vi "itc 503 box controller.vi"(6 "Log File Path":path, 7 "itc box action":T3=enum."read sweep table", 8 "error in":errorcluster, 9 "Sweep Table In":dbl[][](array[numeric])=[[650.0, 1334.0, 30.0], [300.0, 1334.0, 0.0], [0.0, 0.0, 0.0], [0.0, 0.0, 0.0], [0.0, 0.0, 0.0], [0.0, 0.0, 0.0], [0.0, 0.0, 0.0], [0.0, 0.0, 0.0], [0.0, 0.0, 0.0], [0.0, 0.0, 0.0], [0.0, 0.0, 0.0], [300.0, 0.0, 0.0], [0.0, 0.0, 0.0], [0.0, 0.0, 0.0], [0.0, 0.0, 0.0], [300.0, 0.0, 0.0]], 10 "input":dbl=300.0, 11 "VISA resource name":refnum<visa-resource-name>="GPIB0::23::INSTR") -> (0 "error out":errorcluster, 1 "Sweep Table":dbl[][](array[numeric])=[[650.0, 1334.0, 30.0], [300.0, 1334.0, 0.0], [0.0, 0.0, 0.0], [0.0, 0.0, 0.0], [0.0, 0.0, 0.0], [0.0, 0.0, 0.0], [0.0, 0.0, 0.0], [0.0, 0.0, 0.0], [0.0, 0.0, 0.0], [0.0, 0.0, 0.0], [0.0, 0.0, 0.0], [300.0, 0.0, 0.0], [0.0, 0.0, 0.0], [0.0, 0.0, 0.0], [0.0, 0.0, 0.0], [300.0, 0.0, 0.0]], 2 "itc box state OUT":T2={"ITC503 Address"="GPIB0::15::INSTR", "ITC temperature"=0.0, "ITC set temperature"=300.0, "heater"=300.0, "gas flow"=1.6, "P"=0.0, "D"=10.0, "I"=0.1, "ITC state"="X0A1C2S01H1L0\r", "nonzero temperature"=0.0, "Magn Field (T)"=0.0})   [LabVIEW 2014]
uses:
  itc 503 box - control.ctl
  itc 503 box state.ctl
  ITC Panel.ctl
  Q - not nan -- real.vi
panel:
  out "F-format string":string
  in  "ITC 503 front panel":T1={"Locked"=FALSE, "Unlocked"=FALSE, "Remote"=FALSE, "Local"=FALSE, "in sweep"=FALSE, "start/stop sweep"=FALSE, "Sweep indicator"="X0A1C2S01H1L0\r", "heater MANUAL"=FALSE, "heater AUTO"=FALSE, "ITC state"="X0A1C2S01H1L0\r", "gas MANUAL"=FALSE, "gas AUTO"=FALSE, "heater"=13.5, "gas flow %"=0.0} {"gas flow %" format="%.3g"; "heater" format="%.3g"}
  out "enabled state":enum16{"disabled", "enabled"}(ring)
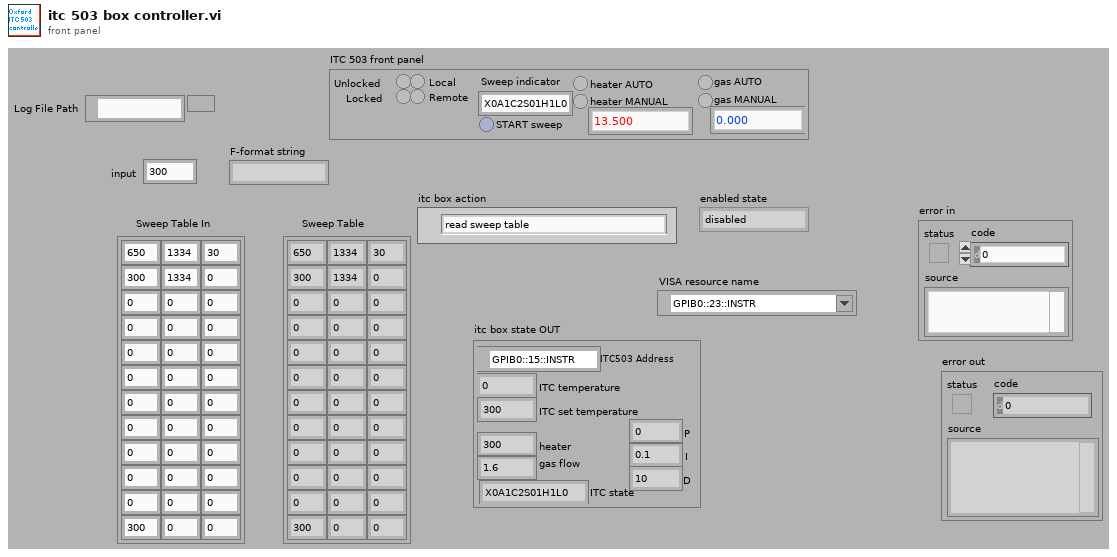
[diagram p1: front panel]
types:
  T1 = typedef "ITC Panel.ctl" = cluster{"Locked":bool, "Unlocked":bool, "Remote":bool, "Local":bool, "in sweep":bool, "start/stop sweep":bool, "Sweep indicator":string, "heater MANUAL":bool, "heater AUTO":bool, "ITC state":string, "gas MANUAL":bool, "gas AUTO":bool, "heater":dbl, "gas flow %":dbl}
  T2 = typedef "itc 503 box state.ctl" = cluster{"ITC503 Address":refnum<visa-resource-name>, "ITC temperature":dbl, "ITC set temperature":dbl, "heater":dbl, "gas flow":dbl, "P":dbl, "D":dbl, "I":dbl, "ITC state":string, "nonzero temperature":dbl, "Magn Field (T)":dbl}
  T3 = typedef "itc 503 box - control.ctl" = enum16{"heater manual and zero", "heater auto", "upload D", "upload I", "upload P", "shut off", "init", "read sweep table", "disable", "enable", "read state", "set gas to", "stop sweep", "start sweep", "test", "set temperature to", "write sweep table", "-void"}
  T4 = enum16{"parse", "start sweep", "stop sweep", "heater auto", "heater manual", "set heater"}
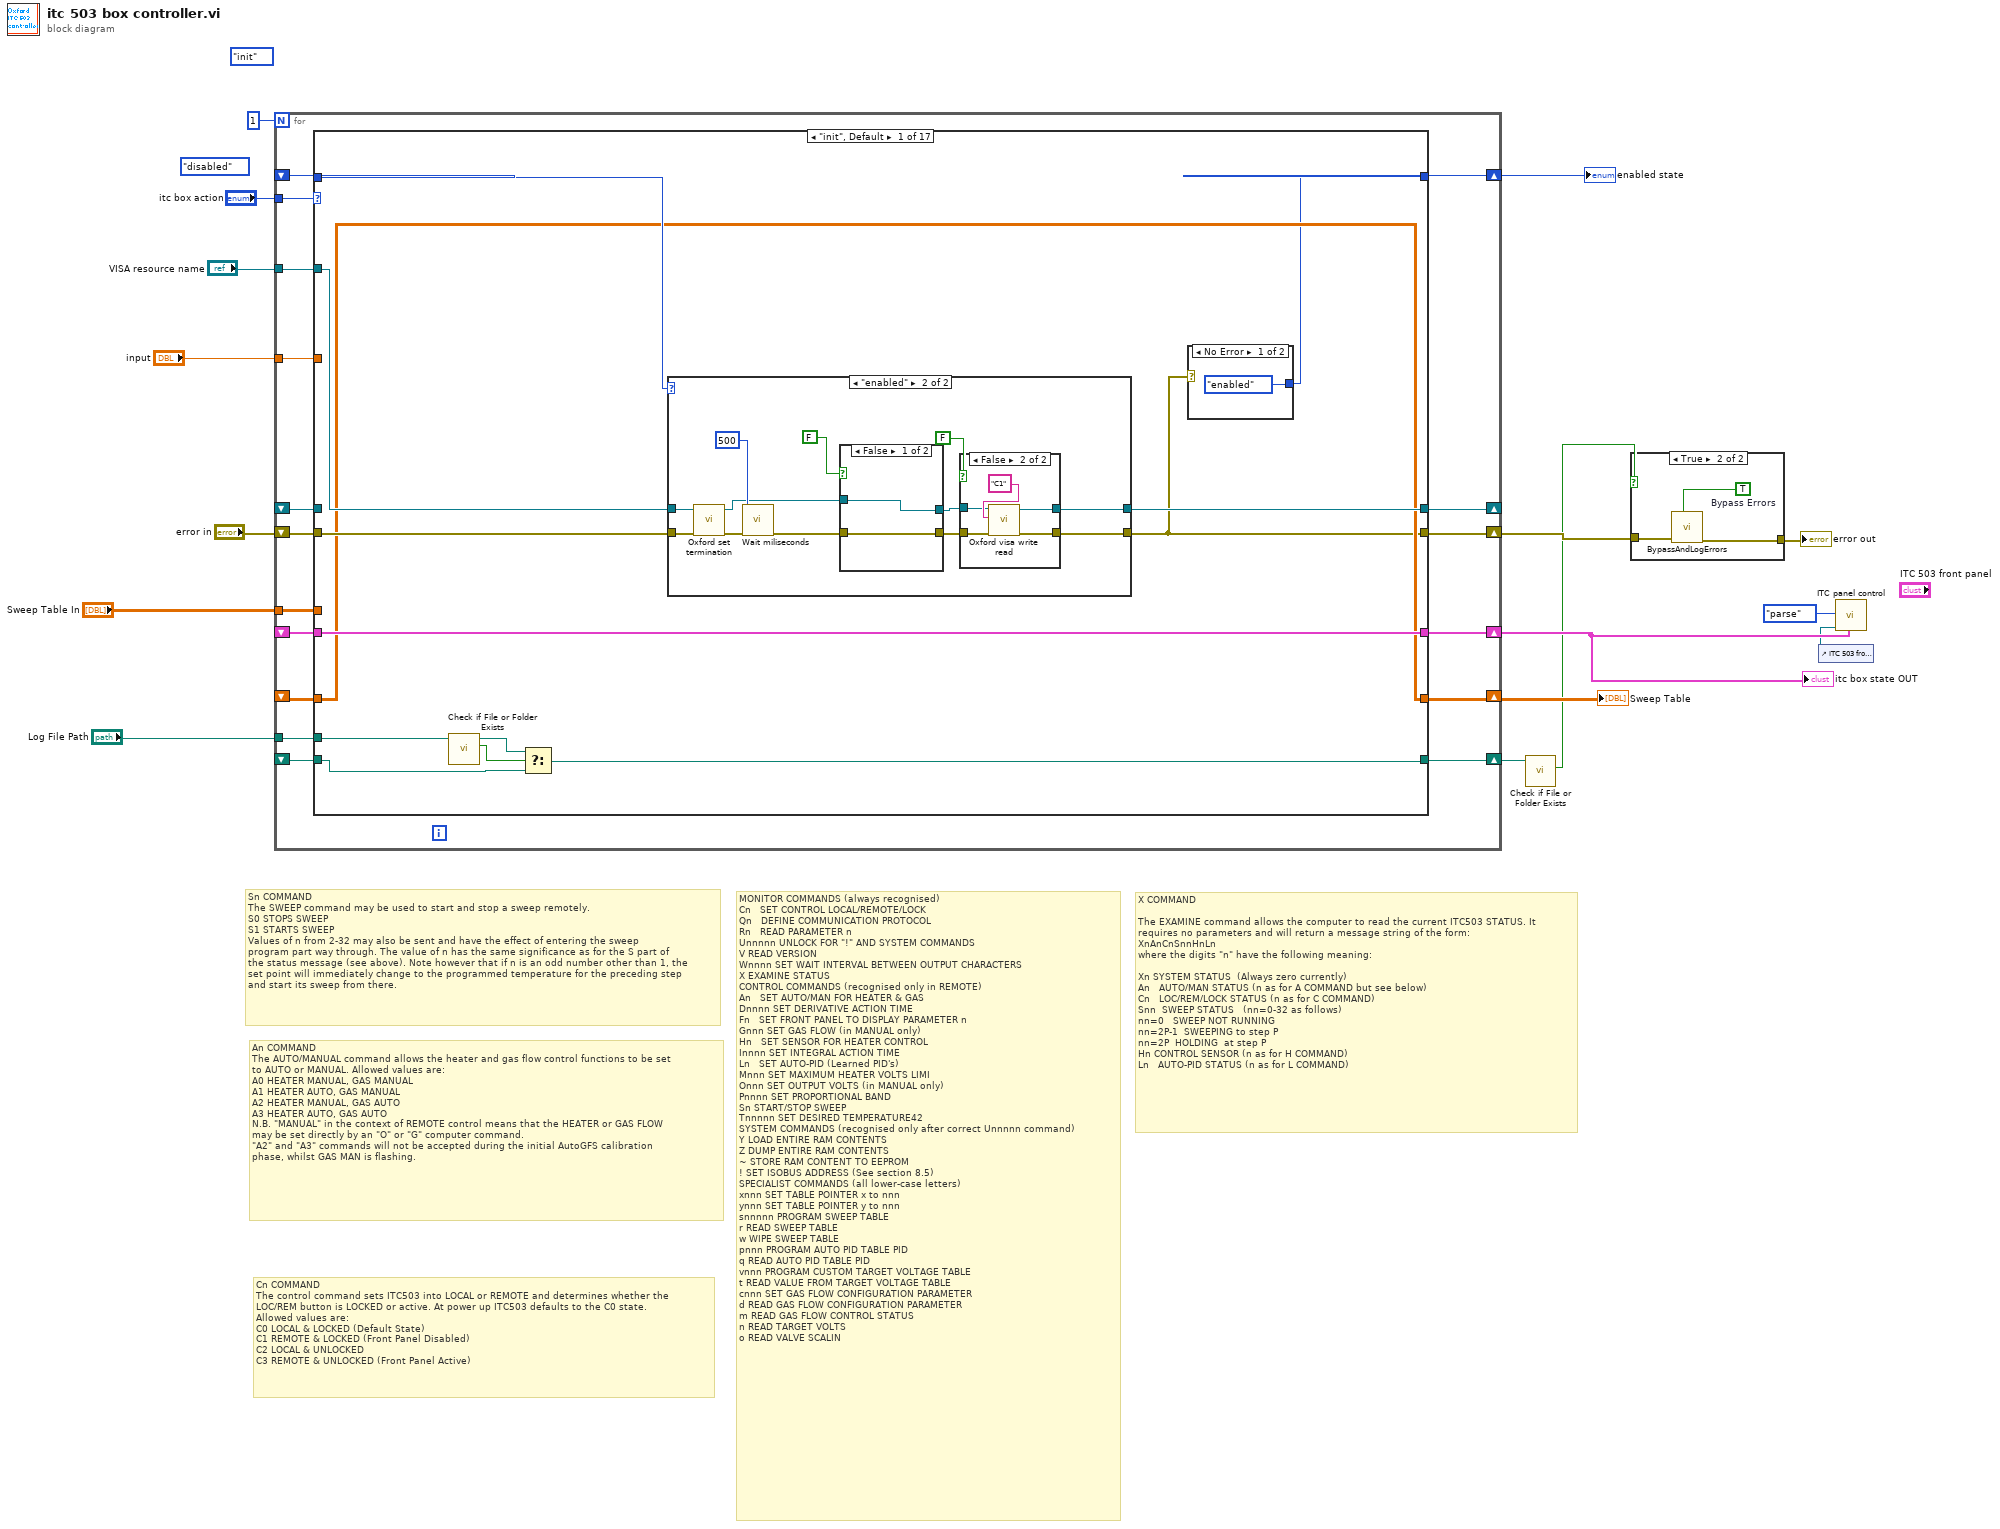
[diagram p0: block diagram]
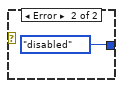
[diagram p3: hidden frame]
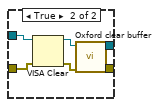
[diagram p5: hidden frame]
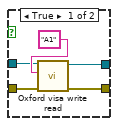
[diagram p6: hidden frame]
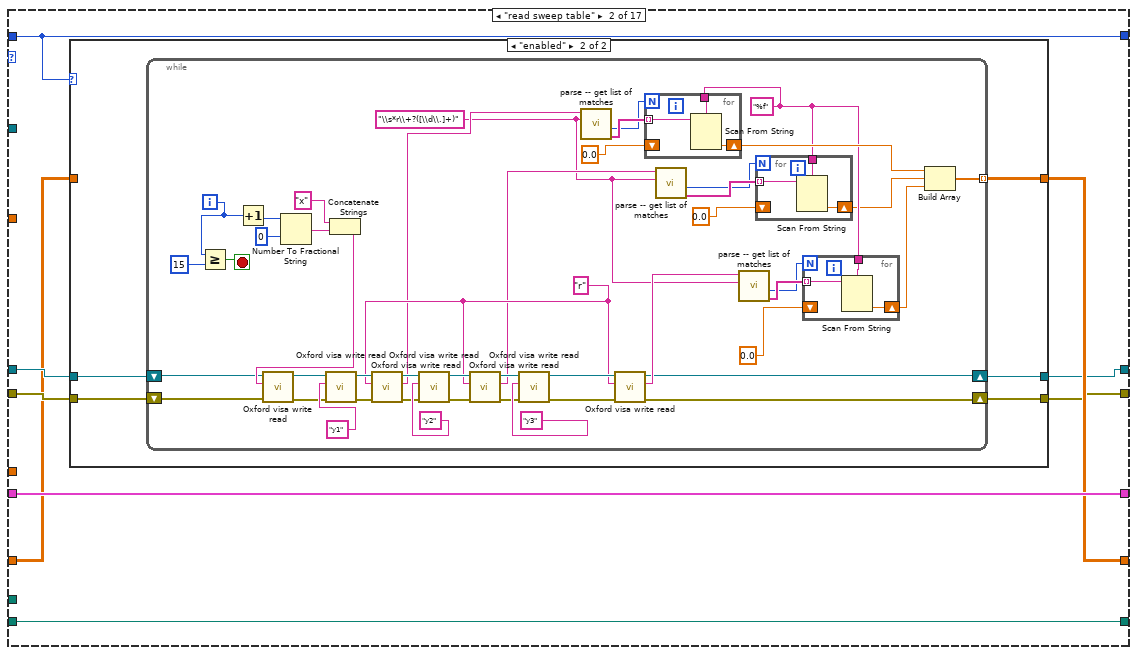
[diagram p7: hidden frame]
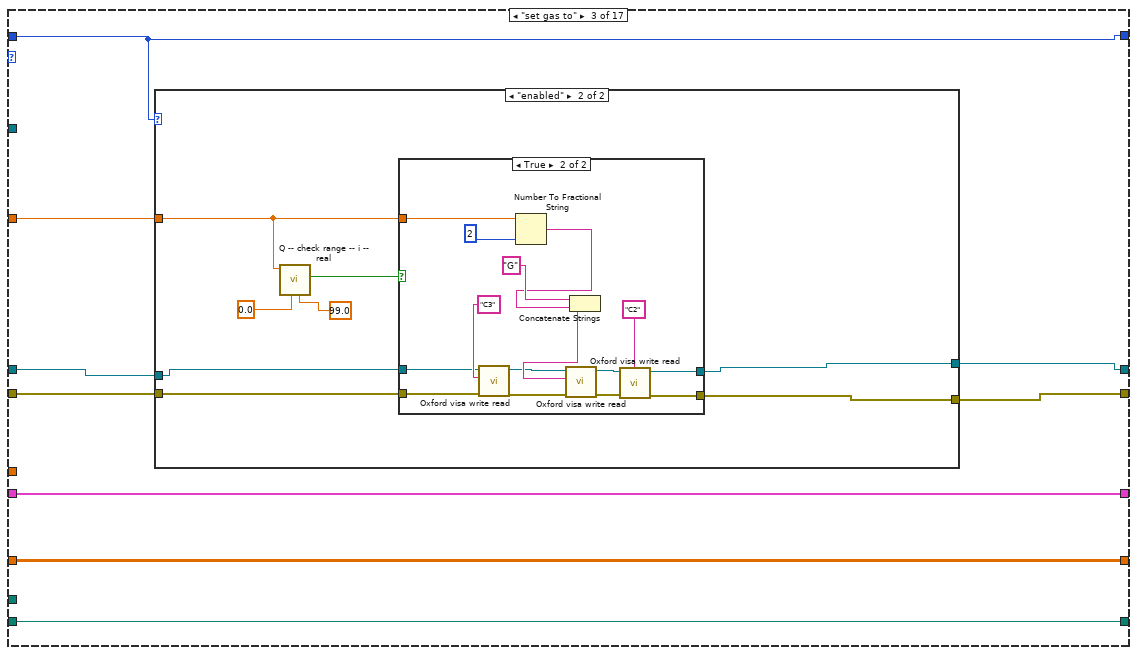
[diagram p9: hidden frame]
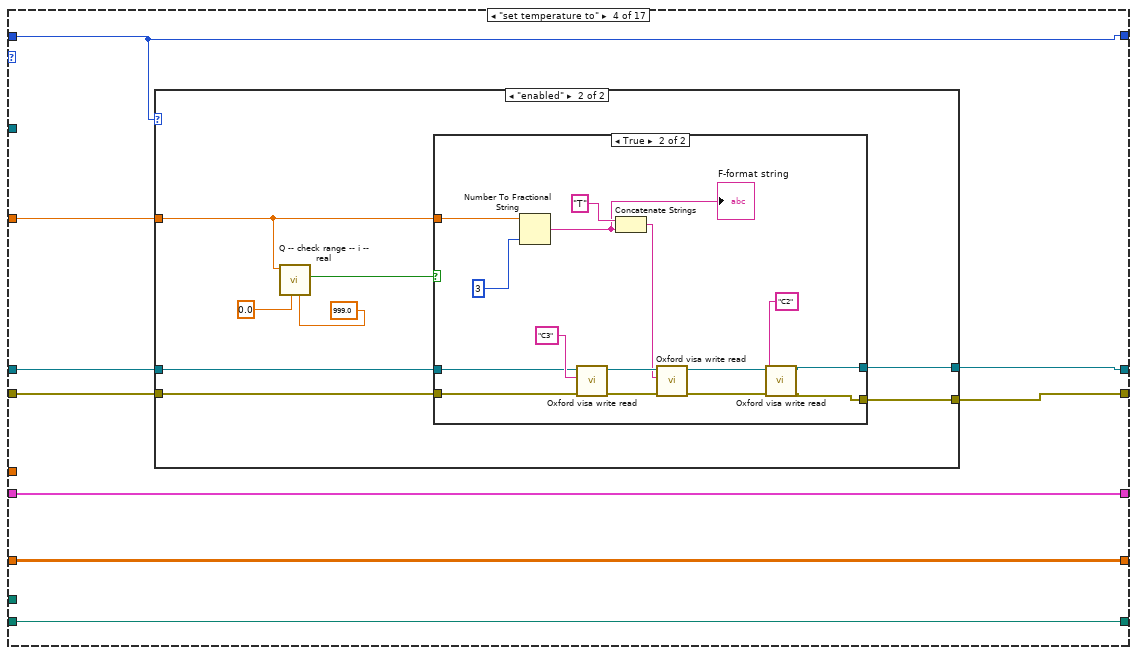
[diagram p12: hidden frame]
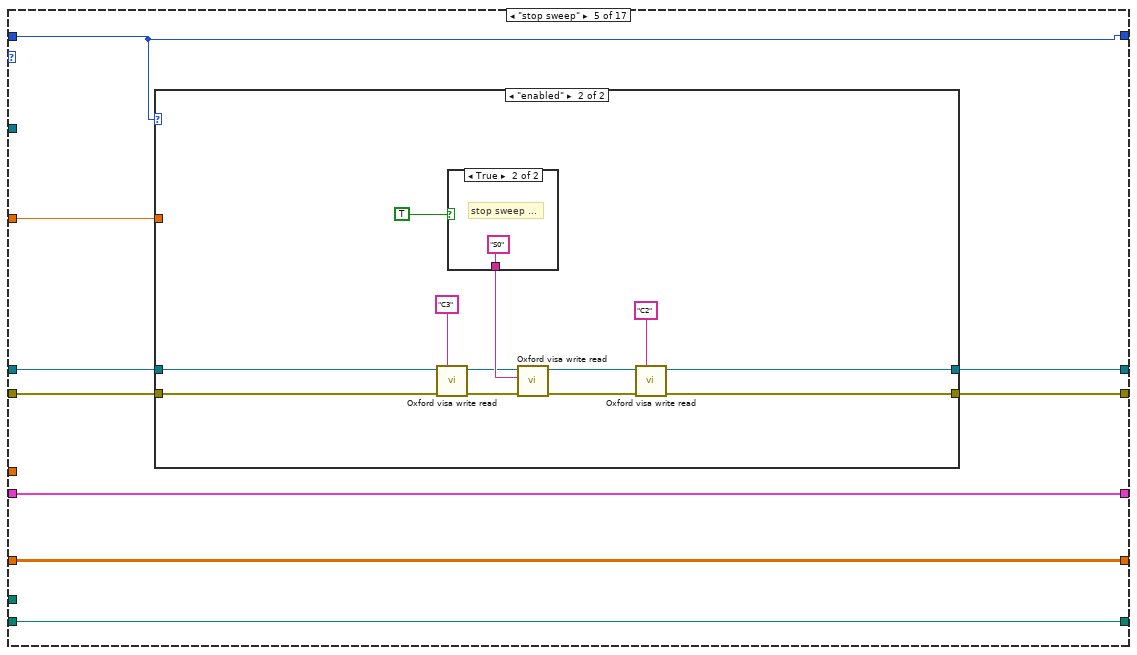
[diagram p15: hidden frame]
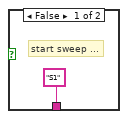
[diagram p17: hidden frame]
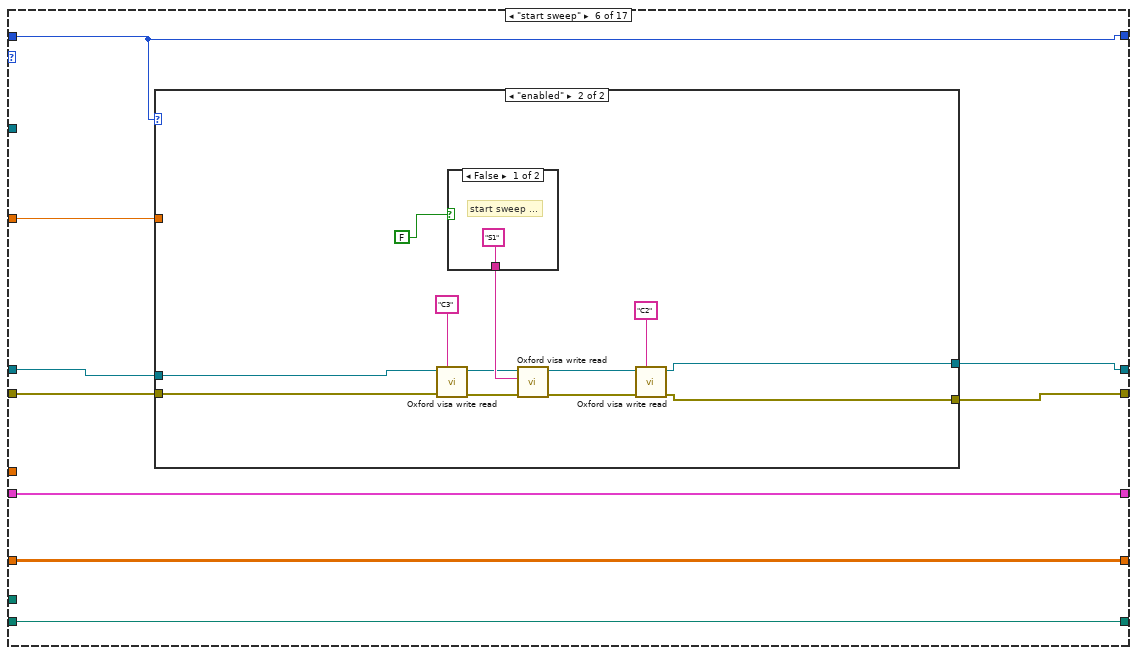
[diagram p18: hidden frame]
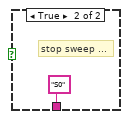
[diagram p20: hidden frame]
diagram:
  (unwired) enum16{"disabled", "enabled"}."disabled" ("disable interaction with itc  2")
  (unwired) itc_503_box_-_control."init" ("itc box action")
  # "Cn COMMAND\nThe control command sets ITC503 into LOCAL or REMOTE and determines whether the\nLOC/REM button is LOCKED or active. At power up ITC503 defaults to the C0 state.\nAllowed values are:\nC0 LOCAL & LOCKED (Default State)\nC1 REMOTE & LOCKED (Front Panel Disabled)\nC2 LOCAL & UNLOCKED\nC3 REMOTE & UNLOCKED (Front Panel Active)"
  # "An COMMAND\nThe AUTO/MANUAL command allows the heater and gas flow control functions to be set\nto AUTO or MANUAL. Allowed values are:\nA0 HEATER MANUAL, GAS MANUAL\nA1 HEATER AUTO, GAS MANUAL\nA2 HEATER MANUAL, GAS AUTO\nA3 HEATER AUTO, GAS AUTO\nN.B. \"MANUAL\" in the context of REMOTE control means that the HEATER or GAS FLOW\nmay be set directly by an \"O\" or \"G\" computer command.\n\"A2\" and \"A3\" commands will not be accepted during the initial AutoGFS calibration\nphase, whilst GAS MAN is flashing."
  # "MONITOR COMMANDS (always recognised)\nCn   SET CONTROL LOCAL/REMOTE/LOCK\nQn   DEFINE COMMUNICATION PROTOCOL\nRn   READ PARAMETER n\nUnnnnn UNLOCK FOR \"!\" AND SYSTEM COMMANDS\nV READ VERSION\nWnnnn SET WAIT INTERVAL BETWEEN OUTPUT CHARACTERS\nX EXAMINE STATUS\nCONTROL COMMANDS (recognised only in REMOTE)\nAn   SET AUTO/MAN FOR HEATER & GAS\nDnnnn SET DERIVATIVE ACTION TIME\nFn   SET FRONT PANEL TO DISPLAY PARAMETER n\nGnnn SET GAS FLOW (in MANUAL only)\nHn   SET SENSOR FOR HEATER CONTROL\nInnnn SET INTEGRAL ACTION TIME\nLn   SET AUTO-PID (Learned PID's)\nMnnn SET MAXIMUM HEATER VOLTS LIMI\nOnnn SET OUTPUT VOLTS (in MANUAL only)\nPnnnn SET PROPORTIONAL BAND\nSn START/STOP SWEEP\nTnnnnn SET DESIRED TEMPERATURE42\nSYSTEM COMMANDS (recognised only after correct Unnnnn command)\nY LOAD ENTIRE RAM CONTENTS\nZ DUMP ENTIRE RAM CONTENTS\n~ STORE RAM CONTENT TO EEPROM\n! SET ISOBUS ADDRESS (See section 8.5)\nSPECIALIST COMMANDS (all lower-case letters)\nxnnn SET TABLE POINTER x to nnn\nynnn SET TABLE POINTER y to nnn\nsnnnnn PROGRAM SWEEP TABLE\nr READ SWEEP TABLE\nw WIPE SWEEP TABLE\npnnn PROGRAM AUTO PID TABLE PID\nq READ AUTO PID TABLE PID\nvnnn PROGRAM CUSTOM TARGET VOLTAGE TABLE\nt READ VALUE FROM TARGET VOLTAGE TABLE\ncnnn SET GAS FLOW CONFIGURATION PARAMETER\nd READ GAS FLOW CONFIGURATION PARAMETER\nm READ GAS FLOW CONTROL STATUS\nn READ TARGET VOLTS\no READ VALVE SCALIN"
  # "X COMMAND\n\nThe EXAMINE command allows the computer to read the current ITC503 STATUS. It\nrequires no parameters and will return a message string of the form:\nXnAnCnSnnHnLn\nwhere the digits \"n\" have the following meaning:\n\nXn SYSTEM STATUS  (Always zero currently)\nAn   AUTO/MAN STATUS (n as for A COMMAND but see below)\nCn   LOC/REM/LOCK STATUS (n as for C COMMAND)\nSnn  SWEEP STATUS   (nn=0-32 as follows)\nnn=0   SWEEP NOT RUNNING\nnn=2P-1  SWEEPING to step P\nnn=2P  HOLDING  at step P\nHn CONTROL SENSOR (n as for H COMMAND)\nLn   AUTO-PID STATUS (n as for L COMMAND)"
  # "Sn COMMAND\nThe SWEEP command may be used to start and stop a sweep remotely.\nS0 STOPS SWEEP\nS1 STARTS SWEEP\nValues of n from 2-32 may also be sent and have the effect of entering the sweep\nprogram part way through. The value of n has the same significance as for the S part of\nthe status message (see above). Note however that if n is an odd number other than 1, the\nset point will immediately change to the programmed temperature for the preceding step\nand start its sweep from there."
  n1 = for {
    N: 1 -> [_]
    tunnel: "itc box action" -> [w33]
    shift-right: [w31] -> _
    shift-left: _ -> [w32]
    tunnel: "VISA resource name" -> [w30]
    shift-right: [w29] -> w9
    shift-left: _ -> [w28]
    shift-right: [w27] -> w7
    shift-left: _ -> [w25]
    shift-right: [w20] -> w4
    shift-left: "error in" -> [w26]
    shift-right: [w24] -> w12
    shift-left: _ -> [w23]
    tunnel: "input" -> [w22]
    tunnel: "Sweep Table In" -> [w21]
    tunnel: "Log File Path" -> [w19]
    shift-right: [w18] -> w2
    shift-left: _ -> [w17]
    n2 = case shown="\"init\", Default" w33 {
      tunnel: w32 -> [_ w87 w160 w196 w232 w257 w282 w308 w334 w360 w382 w407 w451 w463 w480 w544 w550]
      tunnel: [w46 w84 w157 w193 w229 w254 w279 w305 w331 w357 w379 w404 w451 w460 w477 w544 w550] -> w31
      tunnel: w30 -> [w45 _ _ _ _ _ _ _ _ _ _ _ _ _ _ _ _]
      tunnel: [w39 w83 w154 w190 w226 w251 w276 w302 w328 w354 w376 w401 w452 w457 w476 enum16{"disabled", "enabled"}."disabled" ("disable interaction with itc  2") enum16{"disabled", "enabled"}."enabled" ("disable interaction with itc  2")] -> w29
      tunnel: w28 -> [w44 w83 w154 w190 w226 w251 w276 w302 w328 w354 w376 w401 w452 w457 w476 _ _]
      tunnel: [w42 w89 w156 w192 w228 w253 w278 w304 w330 w356 w378 w403 w454 w459 w481 w542 w548] -> w27
      tunnel: w26 -> [w43 w86 w159 w195 w231 w256 w281 w307 w333 w359 w381 w406 w450 w462 w479 w543 w549]
      tunnel: [w40 w85 w158 w194 w230 w255 w280 w306 w332 w358 w380 w405 w450 w461 w478 w543 w549] -> w20
      tunnel: w25 -> [w42 w89 w156 w192 w228 w253 w278 w304 w330 w356 w378 w403 w454 w459 w475 w542 w548]
      tunnel: [w41 w88 w155 w191 w227 w252 w277 w303 w329 w355 w377 w402 w453 w458 w474 w541 w547] -> w24
      tunnel: w23 -> [w41 w82 w155 w191 w227 w252 w277 w303 w329 w355 w377 w402 w453 w458 w474 w541 w547]
      tunnel: w22 -> [_ _ w161 w197 w233 w258 w283 w309 w335 w361 w383 w408 _ w464 _ _ _]
      tunnel: w21 -> [_ _ _ _ _ _ _ _ _ _ _ _ _ w456 _ _ _]
      tunnel: w19 -> [w38 _ _ _ _ _ _ _ _ _ _ _ _ _ _ _ _]
      tunnel: [w35 w81 w153 w189 w225 w250 w275 w301 w327 w353 w375 w400 w449 w455 w473 w540 w546] -> w18
      tunnel: w17 -> [w34 w81 w153 w189 w225 w250 w275 w301 w327 w353 w375 w400 w449 w455 w473 w540 w546]
      frame "init", Default {
        n3 = call <vilib>:"Check if File or Folder Exists.vi"("path"=w38) -> ("file or folder exists?"=w37:bool, "dup path"=w36:path)  [unwired: 8 in, 1 out]
        n4 = Select(t=w36, s=w37, f=w34) -> (s? t:f=w35:path)
        n5 = case shown="\"enabled\"" w44 {
          tunnel: [w50 w59] -> w46
          tunnel: w45 -> [w50 w56]
          tunnel: w43 -> [w49 w55]
          tunnel: [w49 w58] -> w40
          frame "disabled", Default {
          }
          frame "enabled" {
            n6 = call "Oxford set termination.vi"("error in (no error)"=w55, "VISA resource name"=w56) -> ("error out"=w52:errorcluster, "VISA resource name out"=w51:refnum<visa-resource-name>)  [unwired: 8 in]
            n7 = call "Wait miliseconds.vi"("error in (no error)"=w52, "milliseconds to wait"=u32 500) -> ("error out"=w54:errorcluster)  [unwired: 8 in, 1 out]
            n8 = case shown="False" FALSE {
              tunnel: [w63 w70] -> w62
              tunnel: [w64 w69] -> w61
              tunnel: w54 -> [w63 w65]
              tunnel: w51 -> [w64 w68]
              frame False {
              }
              frame True {
                n9 = VISA Clear(VISA resource name=w68, error in (no error)=w65) -> (VISA resource name out=w67:refnum<visa-resource-name>, error out=w66:errorcluster)
                n10 = call "Oxford clear buffer.vi"("error in (no error)"=w66, "VISA resource name"=w67) -> ("error out"=w70:errorcluster, "VISA resource name out"=w69:refnum<visa-resource-name>)  [unwired: 6 in, 2 out]
              }
            }
            n11 = case shown="False" FALSE {
              tunnel: w62 -> [w74 w79]
              tunnel: w61 -> [w73 w78]
              tunnel: [w72 w77] -> w59
              tunnel: [w71 w76] -> w58
              frame True {
                n12 = call "Oxford visa write read.vi"("error in (no error)"=w74, "write buffer"="A1" ("Command"), "VISA resource name"=w73) -> ("error out"=w71:errorcluster, "VISA resource name out"=w72:refnum<visa-resource-name>)  [unwired: 6 in, 1 out]
              }
              frame False {
                n13 = call "Oxford visa write read.vi"("error in (no error)"=w79, "write buffer"="C1" ("Command"), "VISA resource name"=w78) -> ("error out"=w76:errorcluster, "VISA resource name out"=w77:refnum<visa-resource-name>)  [unwired: 6 in, 1 out]
              }
            }
          }
        }
        n14 = case shown="No Error" w40 {
          tunnel: [enum16{"disabled", "enabled"}."enabled" ("disable interaction with itc  2") enum16{"disabled", "enabled"}."disabled" ("disable interaction with itc  2")] -> w39
          frame No Error {
          }
          frame Error {
          }
        }
      }
      frame "read sweep table" {
        n15 = case shown="\"enabled\"" w83 {
          tunnel: [w90 w97] -> w88
          tunnel: w87 -> [w92 w96]
          tunnel: w86 -> [w91 w95]
          tunnel: [w91 w94] -> w85
          tunnel: [w92 w93] -> w84
          tunnel: w82 -> [w90 _]
          frame "disabled", Default {
          }
          frame "enabled" {
            n16 = while {
              tunnel: [w119] -> w97 mode=indexing
              shift-right: [w99] -> w93
              shift-left: w96 -> [w122]
              shift-right: [w98] -> w94
              shift-left: w95 -> [w129]
              i -> [w117]
              stop <- w116 stop-if-true
              w103 = "\\s*r\\+?([\\d\\.]+)" ("format string")
              w102 = "%f" ("format string")
              w121 = "r" ("string")
              n17 = Greater Or Equal?(x=w117, y=15) -> (x >= y?=w116:bool)
              n18 = Increment(x=w117) -> (x+1=w143:i32)
              n19 = Number To Fractional String(number=w143, precision (6)=i16 0) -> (F-format string=w140:string)  [unwired: 2 in]
              n20 = Concatenate Strings("x" ("string"), w140) -> (w139:string)
              n21 = call "Oxford visa write read.vi"("error in (no error)"=w129, "write buffer"=w139, "VISA resource name"=w122) -> ("error out"=w135:errorcluster, "VISA resource name out"=w123:refnum<visa-resource-name>)  [unwired: 6 in, 1 out]
              n22 = call "Oxford visa write read.vi"("error in (no error)"=w135, "write buffer"="y1" ("string"), "VISA resource name"=w123) -> ("error out"=w134:errorcluster, "VISA resource name out"=w124:refnum<visa-resource-name>)  [unwired: 6 in, 1 out]
              n23 = call "Oxford visa write read.vi"("error in (no error)"=w134, "write buffer"=w121, "VISA resource name"=w124) -> ("error out"=w133:errorcluster, "read buffer"=w115:string, "VISA resource name out"=w125:refnum<visa-resource-name>)  [unwired: 6 in]
              n24 = call "Oxford visa write read.vi"("error in (no error)"=w133, "write buffer"="y2" ("string"), "VISA resource name"=w125) -> ("error out"=w132:errorcluster, "VISA resource name out"=w128:refnum<visa-resource-name>)  [unwired: 6 in, 1 out]
              n25 = call "Oxford visa write read.vi"("error in (no error)"=w132, "write buffer"=w121, "VISA resource name"=w128) -> ("error out"=w131:errorcluster, "read buffer"=w104:string, "VISA resource name out"=w127:refnum<visa-resource-name>)  [unwired: 6 in]
              n26 = call "Oxford visa write read.vi"("error in (no error)"=w131, "write buffer"="y3" ("string"), "VISA resource name"=w127) -> ("error out"=w130:errorcluster, "VISA resource name out"=w126:refnum<visa-resource-name>)  [unwired: 6 in, 1 out]
              n27 = call "parse -- get list of matches.vi"("regexp"=w103, "string"=w115) -> ("Array"=w114:string[], "number of free elastic constants"=w113:i32)  [unwired: 7 in, 1 out]
              n28 = call "Oxford visa write read.vi"("error in (no error)"=w130, "write buffer"=w121, "VISA resource name"=w126) -> ("error out"=w98:errorcluster, "read buffer"=w105:string, "VISA resource name out"=w99:refnum<visa-resource-name>)  [unwired: 6 in]
              n29 = for {
                N: w113 -> [_]
                tunnel: w102 -> [w151]
                tunnel: w114 -> [w150] mode=indexing
                shift-right: [w152] -> w120
                shift-left: 0.0 -> [_]
                n30 = Scan From String(format string=w151, input string=w150) -> (output 1=w152:dbl)  [unwired: 3 in, 3 out]
              }
              n31 = call "parse -- get list of matches.vi"("regexp"=w103, "string"=w104) -> ("Array"=w111:string[], "number of free elastic constants"=w110:i32)  [unwired: 7 in, 1 out]
              n32 = call "parse -- get list of matches.vi"("regexp"=w103, "string"=w105) -> ("Array"=w108:string[], "number of free elastic constants"=w107:i32)  [unwired: 7 in, 1 out]
              n33 = for {
                N: w110 -> [_]
                tunnel: w111 -> [w148] mode=indexing
                shift-right: [w149] -> w100
                shift-left: 0.0 -> [_]
                tunnel: w102 -> [w147]
                n34 = Scan From String(format string=w147, input string=w148) -> (output 1=w149:dbl)  [unwired: 3 in, 3 out]
              }
              n35 = for {
                N: w107 -> [_]
                tunnel: w108 -> [w145] mode=indexing
                shift-right: [w146] -> w101
                shift-left: 0.0 -> [_]
                tunnel: w102 -> [w144]
                n36 = Scan From String(format string=w144, input string=w145) -> (output 1=w146:dbl)  [unwired: 3 in, 3 out]
              }
              n37 = Build Array(w120, w100, w101) -> (w119:dbl[])
            }
          }
        }
      }
      frame "set gas to" {
        n38 = case shown="\"enabled\"" w154 {
          tunnel: w161 -> [_ w169]
          tunnel: w160 -> [w163 w167]
          tunnel: w159 -> [w162 w166]
          tunnel: [w162 w165] -> w158
          tunnel: [w163 w164] -> w157
          frame "disabled", Default {
          }
          frame "enabled" {
            n39 = call "Q -- check range -- i -- real.vi"("upper"=99.0, "lower"=0.0, "number"=w169) -> ("in range?"=w168:bool)  [unwired: 6 in, 2 out]
            n40 = case shown="True" w168 {
              tunnel: w166 -> [w173 w180]
              tunnel: [w173 w179] -> w165
              tunnel: [w172 w176] -> w164
              tunnel: w169 -> [_ w175]
              tunnel: w167 -> [w172 w174]
              frame False {
                # "need to rize some kind of error ..."
              }
              frame True {
                n41 = call "Oxford visa write read.vi"("error in (no error)"=w180, "write buffer"="C3" ("Command"), "VISA resource name"=w174) -> ("error out"=w184:errorcluster, "VISA resource name out"=w178:refnum<visa-resource-name>)  [unwired: 6 in, 1 out]
                n42 = Number To Fractional String(number=w175, precision (6)=i16 2) -> (F-format string=w185:string)  [unwired: 2 in]
                n43 = Concatenate Strings("G" ("string"), w185) -> (w182:string)
                n44 = call "Oxford visa write read.vi"("error in (no error)"=w184, "write buffer"=w182, "VISA resource name"=w178) -> ("error out"=w183:errorcluster, "VISA resource name out"=w177:refnum<visa-resource-name>)  [unwired: 6 in, 1 out]
                n45 = call "Oxford visa write read.vi"("error in (no error)"=w183, "write buffer"="C2" ("Command"), "VISA resource name"=w177) -> ("error out"=w179:errorcluster, "VISA resource name out"=w176:refnum<visa-resource-name>)  [unwired: 6 in, 1 out]
              }
            }
          }
        }
      }
      frame "set temperature to" {
        n46 = case shown="\"enabled\"" w190 {
          tunnel: w197 -> [_ w201]
          tunnel: w196 -> [w199 w205]
          tunnel: w195 -> [w198 w200]
          tunnel: [w198 w203] -> w194
          tunnel: [w199 w204] -> w193
          frame "disabled", Default {
          }
          frame "enabled" {
            n47 = call "Q -- check range -- i -- real.vi"("upper"=999.0, "lower"=0.0, "number"=w201) -> ("in range?"=w202:bool)  [unwired: 6 in, 2 out]
            n48 = case shown="True" w202 {
              tunnel: w205 -> [w209 w214]
              tunnel: [w209 w213] -> w204
              tunnel: [w208 w212] -> w203
              tunnel: w201 -> [_ w211]
              tunnel: w200 -> [w208 w210]
              frame False {
              }
              frame True {
                n49 = Number To Fractional String(number=w211, precision (6)=i16 3) -> (F-format string=w219:string)  [unwired: 2 in]
                "F-format string" <- w219
                n50 = call "Oxford visa write read.vi"("error in (no error)"=w210, "write buffer"="C3" ("Command"), "VISA resource name"=w214) -> ("error out"=w224:errorcluster, "VISA resource name out"=w223:refnum<visa-resource-name>)  [unwired: 6 in, 1 out]
                n51 = Concatenate Strings("T" ("Command"), w219) -> (w217:string)
                n52 = call "Oxford visa write read.vi"("error in (no error)"=w224, "write buffer"=w217, "VISA resource name"=w223) -> ("error out"=w215:errorcluster, "VISA resource name out"=w216:refnum<visa-resource-name>)  [unwired: 6 in, 1 out]
                n53 = call "Oxford visa write read.vi"("error in (no error)"=w215, "write buffer"="C2" ("Command"), "VISA resource name"=w216) -> ("error out"=w212:errorcluster, "VISA resource name out"=w213:refnum<visa-resource-name>)  [unwired: 6 in, 1 out]
              }
            }
          }
        }
      }
      frame "stop sweep" {
        n54 = case shown="\"enabled\"" w226 {
          tunnel: w233 -> [_ _]
          tunnel: w232 -> [w235 w236]
          tunnel: w231 -> [w234 w239]
          tunnel: [w234 w238] -> w230
          tunnel: [w235 w237] -> w229
          frame "disabled", Default {
          }
          frame "enabled" {
            n55 = call "Oxford visa write read.vi"("error in (no error)"=w239, "write buffer"="C3" ("Command"), "VISA resource name"=w236) -> ("error out"=w243:errorcluster, "VISA resource name out"=w242:refnum<visa-resource-name>)  [unwired: 6 in, 1 out]
            n56 = case shown="True" TRUE {
              tunnel: ["S1" ("write buffer") "S0" ("write buffer")] -> w247
              frame False {
                # "start sweep ..."
              }
              frame True {
                # "stop sweep ..."
              }
            }
            n57 = call "Oxford visa write read.vi"("error in (no error)"=w243, "write buffer"=w247, "VISA resource name"=w242) -> ("error out"=w246:errorcluster, "VISA resource name out"=w244:refnum<visa-resource-name>)  [unwired: 6 in, 1 out]
            n58 = call "Oxford visa write read.vi"("error in (no error)"=w246, "write buffer"="C2" ("Command"), "VISA resource name"=w244) -> ("error out"=w238:errorcluster, "VISA resource name out"=w237:refnum<visa-resource-name>)  [unwired: 6 in, 1 out]
          }
        }
      }
      frame "start sweep" {
        n59 = case shown="\"enabled\"" w251 {
          tunnel: w258 -> [_ _]
          tunnel: w257 -> [w260 w261]
          tunnel: w256 -> [w259 w264]
          tunnel: [w259 w263] -> w255
          tunnel: [w260 w262] -> w254
          frame "disabled", Default {
          }
          frame "enabled" {
            n60 = call "Oxford visa write read.vi"("error in (no error)"=w264, "write buffer"="C3" ("Command"), "VISA resource name"=w261) -> ("error out"=w268:errorcluster, "VISA resource name out"=w267:refnum<visa-resource-name>)  [unwired: 6 in, 1 out]
            n61 = case shown="False" FALSE {
              tunnel: ["S1" ("write buffer") "S0" ("write buffer")] -> w272
              frame False {
                # "start sweep ..."
              }
              frame True {
                # "stop sweep ..."
              }
            }
            n62 = call "Oxford visa write read.vi"("error in (no error)"=w268, "write buffer"=w272, "VISA resource name"=w267) -> ("error out"=w271:errorcluster, "VISA resource name out"=w269:refnum<visa-resource-name>)  [unwired: 6 in, 1 out]
            n63 = call "Oxford visa write read.vi"("error in (no error)"=w271, "write buffer"="C2" ("Command"), "VISA resource name"=w269) -> ("error out"=w263:errorcluster, "VISA resource name out"=w262:refnum<visa-resource-name>)  [unwired: 6 in, 1 out]
          }
        }
      }
      frame "upload P" {
        n64 = case shown="\"enabled\"" w276 {
          tunnel: w283 -> [_ w286]
          tunnel: w282 -> [w285 w288]
          tunnel: w281 -> [w284 w289]
          tunnel: [w284 w291] -> w280
          tunnel: [w285 w292] -> w279
          frame "disabled", Default {
          }
          frame "enabled" {
            n65 = Number To Fractional String(number=w286, precision (6)=i16 4 ("width (-)")) -> (F-format string=w298:string)  [unwired: 2 in]
            n66 = call "Oxford visa write read.vi"("error in (no error)"=w289, "write buffer"="C3" ("Command"), "VISA resource name"=w288) -> ("error out"=w297:errorcluster, "VISA resource name out"=w294:refnum<visa-resource-name>)  [unwired: 6 in, 1 out]
            n67 = Concatenate Strings("P" ("string"), w298) -> (w300:string)
            n68 = call "Oxford visa write read.vi"("error in (no error)"=w297, "write buffer"=w300, "VISA resource name"=w294) -> ("error out"=w290:errorcluster, "VISA resource name out"=w293:refnum<visa-resource-name>)  [unwired: 6 in, 1 out]
            n69 = call "Oxford visa write read.vi"("error in (no error)"=w290, "write buffer"="C2" ("Command"), "VISA resource name"=w293) -> ("error out"=w291:errorcluster, "VISA resource name out"=w292:refnum<visa-resource-name>)  [unwired: 6 in, 1 out]
          }
        }
      }
      frame "upload I" {
        n70 = case shown="\"enabled\"" w302 {
          tunnel: w309 -> [_ w312]
          tunnel: w308 -> [w311 w314]
          tunnel: w307 -> [w310 w315]
          tunnel: [w310 w317] -> w306
          tunnel: [w311 w318] -> w305
          frame "disabled", Default {
          }
          frame "enabled" {
            n71 = Number To Fractional String(number=w312, precision (6)=i16 4 ("width (-)")) -> (F-format string=w324:string)  [unwired: 2 in]
            n72 = call "Oxford visa write read.vi"("error in (no error)"=w315, "write buffer"="C3" ("Command"), "VISA resource name"=w314) -> ("error out"=w323:errorcluster, "VISA resource name out"=w320:refnum<visa-resource-name>)  [unwired: 6 in, 1 out]
            n73 = Concatenate Strings("I" ("string"), w324) -> (w326:string)
            n74 = call "Oxford visa write read.vi"("error in (no error)"=w323, "write buffer"=w326, "VISA resource name"=w320) -> ("error out"=w316:errorcluster, "VISA resource name out"=w319:refnum<visa-resource-name>)  [unwired: 6 in, 1 out]
            n75 = call "Oxford visa write read.vi"("error in (no error)"=w316, "write buffer"="C2" ("Command"), "VISA resource name"=w319) -> ("error out"=w317:errorcluster, "VISA resource name out"=w318:refnum<visa-resource-name>)  [unwired: 6 in, 1 out]
          }
        }
      }
      frame "upload D" {
        n76 = case shown="\"enabled\"" w328 {
          tunnel: w335 -> [_ w338]
          tunnel: w334 -> [w337 w340]
          tunnel: w333 -> [w336 w341]
          tunnel: [w336 w343] -> w332
          tunnel: [w337 w344] -> w331
          frame "disabled", Default {
          }
          frame "enabled" {
            n77 = Number To Fractional String(number=w338, precision (6)=i16 4 ("width (-)")) -> (F-format string=w350:string)  [unwired: 2 in]
            n78 = call "Oxford visa write read.vi"("error in (no error)"=w341, "write buffer"="C3" ("Command"), "VISA resource name"=w340) -> ("error out"=w349:errorcluster, "VISA resource name out"=w346:refnum<visa-resource-name>)  [unwired: 6 in, 1 out]
            n79 = Concatenate Strings("D" ("string"), w350) -> (w352:string)
            n80 = call "Oxford visa write read.vi"("error in (no error)"=w349, "write buffer"=w352, "VISA resource name"=w346) -> ("error out"=w342:errorcluster, "VISA resource name out"=w345:refnum<visa-resource-name>)  [unwired: 6 in, 1 out]
            n81 = call "Oxford visa write read.vi"("error in (no error)"=w342, "write buffer"="C2" ("Command"), "VISA resource name"=w345) -> ("error out"=w343:errorcluster, "VISA resource name out"=w344:refnum<visa-resource-name>)  [unwired: 6 in, 1 out]
          }
        }
      }
      frame "heater auto" {
        n82 = case shown="\"enabled\"" w354 {
          tunnel: w361 -> [_ _]
          tunnel: w360 -> [w363 w367]
          tunnel: w359 -> [w362 w364]
          tunnel: [w362 w365] -> w358
          tunnel: [w363 w366] -> w357
          frame "disabled", Default {
          }
          frame "enabled" {
            n83 = call "Oxford visa write read.vi"("error in (no error)"=w364, "write buffer"="C3" ("Command"), "VISA resource name"=w367) -> ("error out"=w374:errorcluster, "VISA resource name out"=w372:refnum<visa-resource-name>)  [unwired: 6 in, 1 out]
            n84 = call "Oxford visa write read.vi"("error in (no error)"=w374, "write buffer"="A1" ("Command"), "VISA resource name"=w372) -> ("error out"=w368:errorcluster, "VISA resource name out"=w369:refnum<visa-resource-name>)  [unwired: 6 in, 1 out]
            n85 = call "Oxford visa write read.vi"("error in (no error)"=w368, "write buffer"="C2" ("Command"), "VISA resource name"=w369) -> ("error out"=w365:errorcluster, "VISA resource name out"=w366:refnum<visa-resource-name>)  [unwired: 6 in, 1 out]
          }
        }
      }
      frame "heater manual and zero" {
        n86 = case shown="\"enabled\"" w376 {
          tunnel: w383 -> [_ _]
          tunnel: w382 -> [w385 w389]
          tunnel: w381 -> [w384 w388]
          tunnel: [w384 w387] -> w380
          tunnel: [w385 w386] -> w379
          frame "disabled", Default {
          }
          frame "enabled" {
            n87 = call "Oxford visa write read.vi"("error in (no error)"=w388, "write buffer"="C3" ("Command"), "VISA resource name"=w389) -> ("error out"=w391:errorcluster, "VISA resource name out"=w394:refnum<visa-resource-name>)  [unwired: 6 in, 1 out]
            n88 = call "Oxford visa write read.vi"("error in (no error)"=w391, "write buffer"="A0" ("Command"), "VISA resource name"=w394) -> ("error out"=w390:errorcluster, "VISA resource name out"=w393:refnum<visa-resource-name>)  [unwired: 6 in, 1 out]
            n89 = call "Oxford visa write read.vi"("error in (no error)"=w390, "write buffer"="O000" ("Command"), "VISA resource name"=w393) -> ("error out"=w398:errorcluster, "VISA resource name out"=w397:refnum<visa-resource-name>)  [unwired: 6 in, 1 out]
            n90 = call "Oxford visa write read.vi"("error in (no error)"=w398, "write buffer"="C2" ("Command"), "VISA resource name"=w397) -> ("error out"=w387:errorcluster, "VISA resource name out"=w386:refnum<visa-resource-name>)  [unwired: 6 in, 1 out]
          }
        }
      }
      frame "shut off" {
        n91 = case shown="\"enabled\"" w401 {
          tunnel: w408 -> [_ _]
          tunnel: w407 -> [w410 w420]
          tunnel: w406 -> [w409 w419]
          tunnel: [w409 w418] -> w405
          tunnel: [w410 w417] -> w404
          frame "disabled", Default {
          }
          frame "enabled" {
            w416 = 1.0  # Gas %
            # "stop sweep"
            # "Heater V = 0"
            # "Heater Manual"
            # "Remote"
            n92 = for {
              tunnel: string[] ["C3", "A0", "S0", "O000"] -> [w447] mode=indexing
              shift-right: [w445] -> w415
              shift-left: w420 -> [w448]
              shift-right: [w444] -> w414
              shift-left: w419 -> [w446]
              n93 = call "Oxford visa write read.vi"("error in (no error)"=w446, "write buffer"=w447, "VISA resource name"=w448) -> ("error out"=w444:errorcluster, "VISA resource name out"=w445:refnum<visa-resource-name>)  [unwired: 6 in, 1 out]
            }
            n94 = case shown="True" TRUE {
              tunnel: w414 -> [w423 w430]
              tunnel: [w423 w429] -> w412
              tunnel: [w422 w426] -> w413
              tunnel: w415 -> [w422 w425]
              tunnel: w416 -> [_ w424]
              frame False {
                # "need to rize some kind of error ..."
              }
              frame True {
                n95 = call "Oxford visa write read.vi"("error in (no error)"=w430, "write buffer"="C3" ("Command"), "VISA resource name"=w425) -> ("error out"=w434:errorcluster, "VISA resource name out"=w428:refnum<visa-resource-name>)  [unwired: 6 in, 1 out]
                n96 = Number To Fractional String(number=w424, precision (6)=i16 2) -> (F-format string=w435:string)  [unwired: 2 in]
                n97 = Concatenate Strings("G" ("string"), w435) -> (w432:string)
                n98 = call "Oxford visa write read.vi"("error in (no error)"=w434, "write buffer"=w432, "VISA resource name"=w428) -> ("error out"=w433:errorcluster, "VISA resource name out"=w427:refnum<visa-resource-name>)  [unwired: 6 in, 1 out]
                n99 = call "Oxford visa write read.vi"("error in (no error)"=w433, "write buffer"="C2" ("Command"), "VISA resource name"=w427) -> ("error out"=w429:errorcluster, "VISA resource name out"=w426:refnum<visa-resource-name>)  [unwired: 6 in, 1 out]
              }
            }
            n100 = disable-structure shown="Disabled" {
              disable-tunnel: w413 -> [w442 _]
              disable-tunnel: w412 -> [w441 _]
              disable-tunnel: [w440 _] -> w417
              disable-tunnel: [w439 _] -> w418
              frame Disabled {
                w443 = "C0"  # write buffer
                # "Local locked"
                n101 = call "Oxford visa write read.vi"("error in (no error)"=w441, "write buffer"=w443, "VISA resource name"=w442) -> ("error out"=w439:errorcluster, "VISA resource name out"=w440:refnum<visa-resource-name>)  [unwired: 6 in, 1 out]
              }
              frame Enabled {
              }
            }
          }
        }
      }
      frame "test" {
      }
      frame "write sweep table" {
        n102 = case shown="\"enabled\"" w457 {
          tunnel: w464 -> [_ w467]
          tunnel: w463 -> [w466 w472]
          tunnel: w462 -> [w465 w471]
          tunnel: [w465 w469] -> w461
          tunnel: [w466 w468] -> w460
          tunnel: w456 -> [_ w470]
          frame "disabled", Default {
          }
          frame "enabled" {
            n103 = call "ITC 503 -- upload sweep table.vi"("error in"=w471, "Start set point"=w467, "Sweep Table"=w470, "ITC503 Address"=w472) -> ("error out"=w469:errorcluster, "ITC503 Address OUT"=w468:refnum<visa-resource-name>)  [unwired: 6 in]
          }
        }
      }
      frame "read state" {
        n104 = case shown="\"enabled\"" w476 {
          tunnel: [w482 w490] -> w481
          tunnel: w480 -> [w484 w489]
          tunnel: w479 -> [w483 w488]
          tunnel: [w483 w487] -> w478
          tunnel: [w484 w485] -> w477
          tunnel: w475 -> [w482 _]
          frame "disabled", Default {
          }
          frame "enabled" {
            w506 = FALSE
            n105 = case shown="True" w506 {
              tunnel: [w534 w538] -> w504
              tunnel: [w533 w537] -> w505
              tunnel: w489 -> [w534 w536]
              tunnel: w488 -> [w533 w535]
              frame False {
              }
              frame True {
                n106 = call "Oxford visa write read.vi"("error in (no error)"=w535, "write buffer"="C3" ("Command"), "VISA resource name"=w536) -> ("error out"=w537:errorcluster, "VISA resource name out"=w538:refnum<visa-resource-name>)  [unwired: 6 in, 1 out]
              }
            }
            n107 = call "Oxford visa write read.vi"("error in (no error)"=w505, "write buffer"="X", "VISA resource name"=w504) -> ("error out"=w500:errorcluster, "read buffer"=w491:string, "VISA resource name out"=w501:refnum<visa-resource-name>)  [unwired: 6 in]
            n108 = call "Oxford Read Channel.vi"("error in (no error)"=w500, "Channel #"=1 ("Sensor #"), "VISA resource name"=w501) -> ("error out"=w507:errorcluster, "Data"=w497:dbl, "VISA resource name out"=w513:refnum<visa-resource-name>)  [unwired: 5 in, 1 out]
            n109 = call "Oxford Read Channel.vi"("error in (no error)"=w507, "Channel #"=0 ("Sensor #"), "VISA resource name"=w513) -> ("error out"=w508:errorcluster, "Data"=w496:dbl, "VISA resource name out"=w514:refnum<visa-resource-name>)  [unwired: 5 in, 1 out]
            n110 = call "Oxford Read Channel.vi"("error in (no error)"=w508, "Channel #"=6 ("Sensor #"), "VISA resource name"=w514) -> ("error out"=w509:errorcluster, "Data"=w495:dbl, "VISA resource name out"=w515:refnum<visa-resource-name>)  [unwired: 5 in, 1 out]
            n111 = call "Oxford Read Channel.vi"("error in (no error)"=w509, "Channel #"=7 ("Sensor #"), "VISA resource name"=w515) -> ("error out"=w510:errorcluster, "Data"=w494:dbl, "VISA resource name out"=w516:refnum<visa-resource-name>)  [unwired: 5 in, 1 out]
            n112 = call "Oxford Read Channel.vi"("error in (no error)"=w510, "Channel #"=8 ("Sensor #"), "VISA resource name"=w516) -> ("error out"=w511:errorcluster, "Data"=w493:dbl, "VISA resource name out"=w517:refnum<visa-resource-name>)  [unwired: 5 in, 1 out]
            n113 = call "Oxford Read Channel.vi"("error in (no error)"=w511, "Channel #"=9 ("Sensor #"), "VISA resource name"=w517) -> ("error out"=w512:errorcluster, "Data"=w492:dbl, "VISA resource name out"=w518:refnum<visa-resource-name>)  [unwired: 5 in, 1 out]
            n114 = call "Oxford Read Channel.vi"("error in (no error)"=w512, "Channel #"=10 ("Sensor #"), "VISA resource name"=w518) -> ("error out"=w503:errorcluster, "Data"=w486:dbl, "VISA resource name out"=w502:refnum<visa-resource-name>)  [unwired: 5 in, 1 out]
            n115 = case shown="True" w506 {
              tunnel: w502 -> [w526 w531]
              tunnel: w503 -> [w527 w530]
              tunnel: [w527 w529] -> w487
              tunnel: [w526 w528] -> w485
              frame False {
              }
              frame True {
                n116 = call "Oxford visa write read.vi"("error in (no error)"=w530, "write buffer"="C2" ("Command"), "VISA resource name"=w531) -> ("error out"=w529:errorcluster, "VISA resource name out"=w528:refnum<visa-resource-name>)  [unwired: 6 in, 1 out]
              }
            }
            n117 = Bundle By Name(cluster=T2 {"ITC503 Address"="GPIB0::15::INSTR", "ITC temperature"=0.0, "ITC set temperature"=0.0, "heater"=0.0, "gas flow"=0.0, "P"=0.0, "D"=0.0, "I"=0.0, "ITC state"="", "nonzero temperature"=0.0, "Magn Field (T)"=0.0} ("itc box state OUT"), "ITC503 Address"=w485, "ITC temperature"=w497, "ITC set temperature"=w496, "heater"=w495, "gas flow"=w494, "P"=w493, "D"=w486, "I"=w492, "ITC state"=w491) -> (w490:T2)
          }
        }
      }
      frame "disable" {
      }
      frame "enable" {
      }
    }
  }
  "itc box state OUT" <- w7
  "Sweep Table" <- w12
  "enabled state" <- w9
  n118 = call <vilib>:"Check if File or Folder Exists.vi"("path"=w2) -> ("file or folder exists?"=w1:bool)  [unwired: 8 in, 2 out]
  n119 = case shown="True" w1 {
    tunnel: w4 -> [w552 w554]
    tunnel: [w552 w553] -> w3
    frame False {
    }
    frame True {
      w555 = TRUE  # Bypass Errors
      n120 = call "BypassAndLogErrors.vi"("Bypass Errors"=w555, "error in (no error)"=w554) -> ("error out"=w553:errorcluster)  [unwired: 9 in]
    }
  }
  "error out" <- w3
  n121 = control-ref of="ITC 503 front panel"() -> (w6:refnum<vi>)
  n122 = call "ITC panel control.vi"("itc box state"=w7, "action"=T4."parse", "ITC panel IN"=w6) -> ()  [unwired: 8 in, 1 out]
